vi "io_query_ascii_or_bin_floatArray_with_OPC.vi"(7 "Timeout in (0 = OPC timeout)":i32, 8 "error in":errorcluster caption="error in (no error)", 10 "Query":string, 11 "VISA resource name":refnum<visa-resource-name>) -> (0 "error out":errorcluster, 1 "Array Size":i32, 2 "Numbers out":dbl[](array[numeric]) format="%.2e", 3 "VISA resource name out":refnum<visa-resource-name>)   [LabVIEW 2020, in "Rohde&Schwarz RTx Oscilloscopes.lvlib" / "rsidr_core.lvlib"]
doc: "Queries array of <b>floats</b> with OPC. The numbers can be returned in ASCII format or in binary format. The array is always returned as the most-universal double array.\n- For <b>ASCII</b> format, the array numbers are decoded as comma-separated values.\n- For <b>Binary Format</b>, the numbers are decoded based on the session parameter <b>Bin Float Number Format</b>, usually float 32-bit (REAL,32), swapped endianess (instruments usually use low endian, LabVIEW uses big endian)."
uses:
  rsidr_core.lvlib
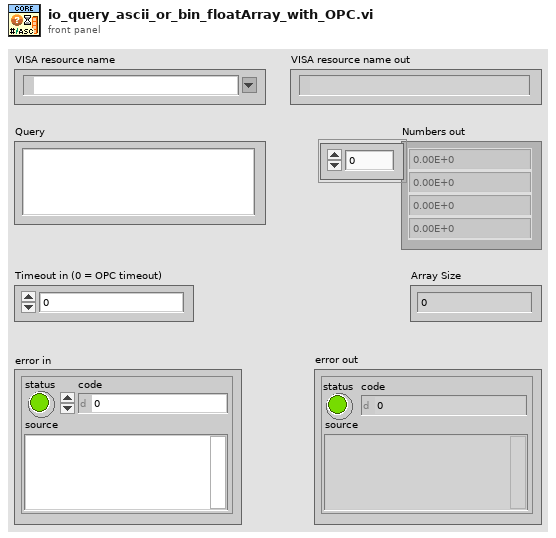
[diagram p1: front panel]
types:
  T1 = typedef "Rohde&Schwarz RTx Oscilloscopes.lvlib/rsidr_core.lvlib/type_Session_Data.ctl" = cluster{"IDN string":string, "Instrument FW":string, "Instr type":string, "Instr type for err. msg.":string, "Installed Options":string[], "Ignore Error Messages":string, "Logging params":variant, "OPC Timeout":i32, "VISA Timeout":i32, "STB Poll VISA Timeout":i32, "Additional Flags":i32, "Wait Before Read":i32, "Wait Before Write":i32, "Option String Flags":i32, "IO Segment Size":i64, "VISA Access Mode":T2, "Interface Type":T3, "OPC Wait Mode":T4, "Bin Float Number  Format":T5, "Bin Integer Number Format":T6, "Simulate":bool, "VXIcapable":bool, "Duplicate Session":bool, "Add LF to Write":bool, "Logging":bool, "Fast Sweep":bool, "Query Instrument Status":bool, "Check Range":bool, "Check Options":bool, "OPC-sync Attr Writes":bool, "OPC-sync Attr Queries":bool}
  T2 = typedef "Rohde&Schwarz RTx Oscilloscopes.lvlib/rsidr_core.lvlib/type_VisaAccessMode.ctl" = u16
  T3 = typedef "Rohde&Schwarz RTx Oscilloscopes.lvlib/rsidr_core.lvlib/type_InterfaceType.ctl" = enum16{"Unknown", "GPIB", "VXI", "GPIB_VXI", "ASRL", "PXI", "TCPIP", "USB", "SOCKET"}
  T4 = typedef "Rohde&Schwarz RTx Oscilloscopes.lvlib/rsidr_core.lvlib/type_OPC_Wait_Mode.ctl" = enum16{"STBpolling", "STBpollingSlow", "STBpollingSuperSlow", "ServiceRequest", "OPCquery"}
  T5 = typedef "Rohde&Schwarz RTx Oscilloscopes.lvlib/rsidr_core.lvlib/type_Binary_Float_Number_Format.ctl" = enum16{"Float_4_Bytes_Swapped", "Float_4_Bytes", "Double_8_Bytes_Swapped", "Double_8_Bytes"}
  T6 = typedef "Rohde&Schwarz RTx Oscilloscopes.lvlib/rsidr_core.lvlib/type_Binary_Integer_Number_Format.ctl" = enum16{"Int32_4_Bytes_Swapped", "Int32_4 Bytes", "Int16_2_Bytes_Swapped", "Int16_2_Bytes"}
  T7 = typedef "Rohde&Schwarz RTx Oscilloscopes.lvlib/rsidr_core.lvlib/type_Attribute.ctl" = cluster{"Identifier":string, "Descriptive Name":string, "Data Type":T8, "Command":string, "Access":T9, "Range Table":string, "Read Callback":string, "Write Callback":string, "Supported Models":string, "Instrument Options":string, "Index":i32, "OPC Wait":bool, "No Status Check":bool, "Cache Only":bool}
  T8 = typedef "Rohde&Schwarz RTx Oscilloscopes.lvlib/rsidr_core.lvlib/type_Attribute_Data_Type.ctl" = enum16{"Integer 32", "Double", "String", "Boolean", "None", "Integer 64", "RawString"}
  T9 = typedef "Rohde&Schwarz RTx Oscilloscopes.lvlib/rsidr_core.lvlib/type_ReadWriteAccess.ctl" = enum16{"Read Only", "Write Only", "Read/Write"}
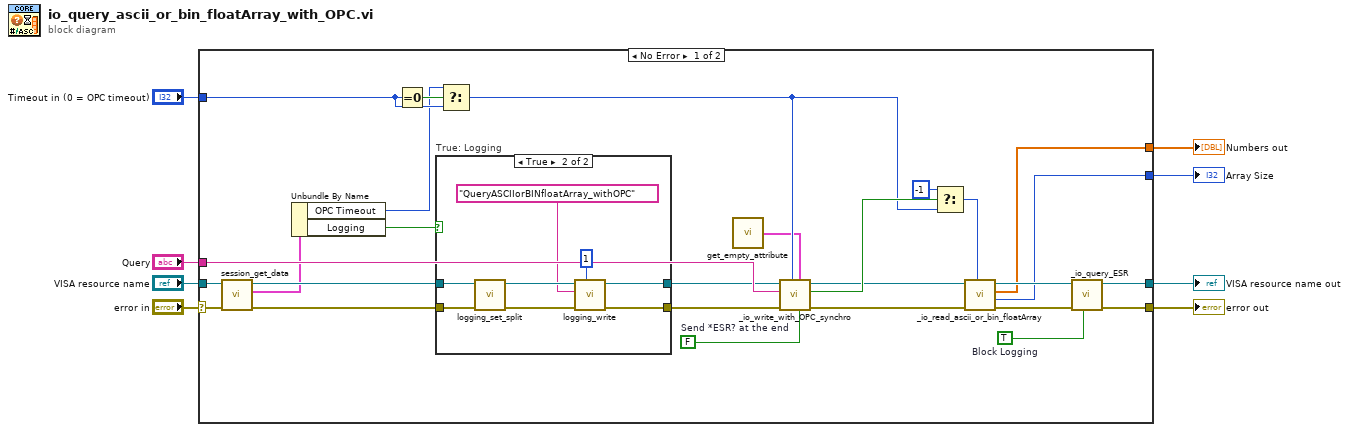
[diagram p0: block diagram]
diagram:
  n1 = case shown="No Error" "error in" {
    selector: "error in" -> [w33 w47]
    tunnel: [w25 w46] -> w8
    tunnel: [w26 w47] -> w7
    tunnel: "VISA resource name" -> [w32 w46]
    tunnel: [w11 _] -> w3
    tunnel: "Query" -> [w35 _]
    tunnel: "Timeout in (0 = OPC timeout)" -> [w20 _]
    tunnel: [w10 _] -> w1
    frame No Error {
      w24 = TRUE  # Block Logging
      w23 = FALSE  # Send *ESR? at the end
      n2 = call "session_get_data.vi"("error in"=w33, "VISA resource name"=w32) -> ("error out"=w31:errorcluster, "Session User Data out"=w29:T1, "VISA resource name out"=w30:refnum<visa-resource-name>)  [unwired: 6 in, 1 out]
      n3 = Unbundle By Name(w29) -> ("OPC Timeout"=w18:i32, "Logging"=w27:bool)
      n4 = Equal To 0?(x=w20) -> (x = 0?=w21:bool)
      n5 = case "True: Logging" shown="True" w27 {
        tunnel: [w36 w41] -> w28
        tunnel: w30 -> [w37 w44]
        tunnel: [w37 w40] -> w34
        tunnel: w31 -> [w36 w39]
        frame False {
        }
        frame True {
          n6 = call "logging_set_split.vi"("error in"=w39, "VISA resource name"=w44) -> ("error out"=w43:errorcluster, "VISA resource name out"=w42:refnum<visa-resource-name>)  [unwired: 8 in]
          n7 = call "logging_write.vi"("Add call chain offset\n(No call chain)"=1 ("Add call chain offset\n(No call chain)"), "error in"=w43, "String to write"="QueryASCIIorBINfloatArray_withOPC" ("format string"), "VISA resource name"=w42) -> ("error out"=w41:errorcluster, "VISA resource name out"=w40:refnum<visa-resource-name>)  [unwired: 6 in]
        }
      }
      n8 = Select(t=w18, s=w21, f=w20) -> (s? t:f=w19:i32)
      n9 = call "get_empty_attribute.vi"() -> ("Empty Attribute out"=w9:T7)
      n10 = call "_io_write_with_OPC_synchro.vi"("Send *ESR? at the end (T)"=w23, "Attribute"=w9, "Timeout in (0 = OPC timeout)"=w19, "error in"=w28, "Write Command"=w35, "VISA resource name"=w34) -> ("error out"=w15:errorcluster, "OPC Waited"=w22:bool, "VISA resource name out"=w14:refnum<visa-resource-name>)  [unwired: 3 in]
      n11 = Select(t=-1, s=w22, f=w19) -> (s? t:f=w16:i32)
      n12 = call "_io_read_ascii_or_bin_floatArray.vi"("Timeout for chunked touts (-1: No chunked touts)"=w16, "error in"=w15, "VISA resource name"=w14) -> ("error out"=w13:errorcluster, "Array Size"=w10:i32, "Numbers out"=w11:dbl[], "VISA resource name out"=w12:refnum<visa-resource-name>)  [unwired: 5 in]
      n13 = call "_io_query_ESR.vi"("Block Logging (F)"=w24, "error in"=w13, "VISA resource name"=w12) -> ("error out"=w26:errorcluster, "VISA resource name out"=w25:refnum<visa-resource-name>)  [unwired: 6 in, 1 out]
    }
    frame Error {
    }
  }
  "error out" <- w7
  "VISA resource name out" <- w8
  "Numbers out" <- w3
  "Array Size" <- w1
